vi "Update Connection Control.vi"(7 "Direction to Include":T1=enum."Publisher", 8 "error in (no error)":errorcluster, 10 "Channels":refnum<vi>, 11 "Channel Connection":refnum<vi>) -> (0 "error out":errorcluster)   [LabVIEW 2021, in "CIF_UI.lvclass"]
uses:
  CIF_UI.lvclass
  Typedef/Channel Connection.ctl
  Typedef/Direction to Include.ctl
  CIF_UI.lvclass/CIF_UI.ctl
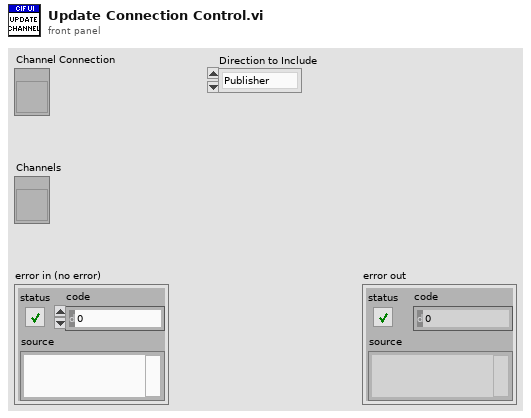
[diagram p1: front panel]
types:
  T1 = typedef "CIF_UI.lvclass/Direction to Include.ctl" = enum16{"All", "Subscriber", "Publisher"}
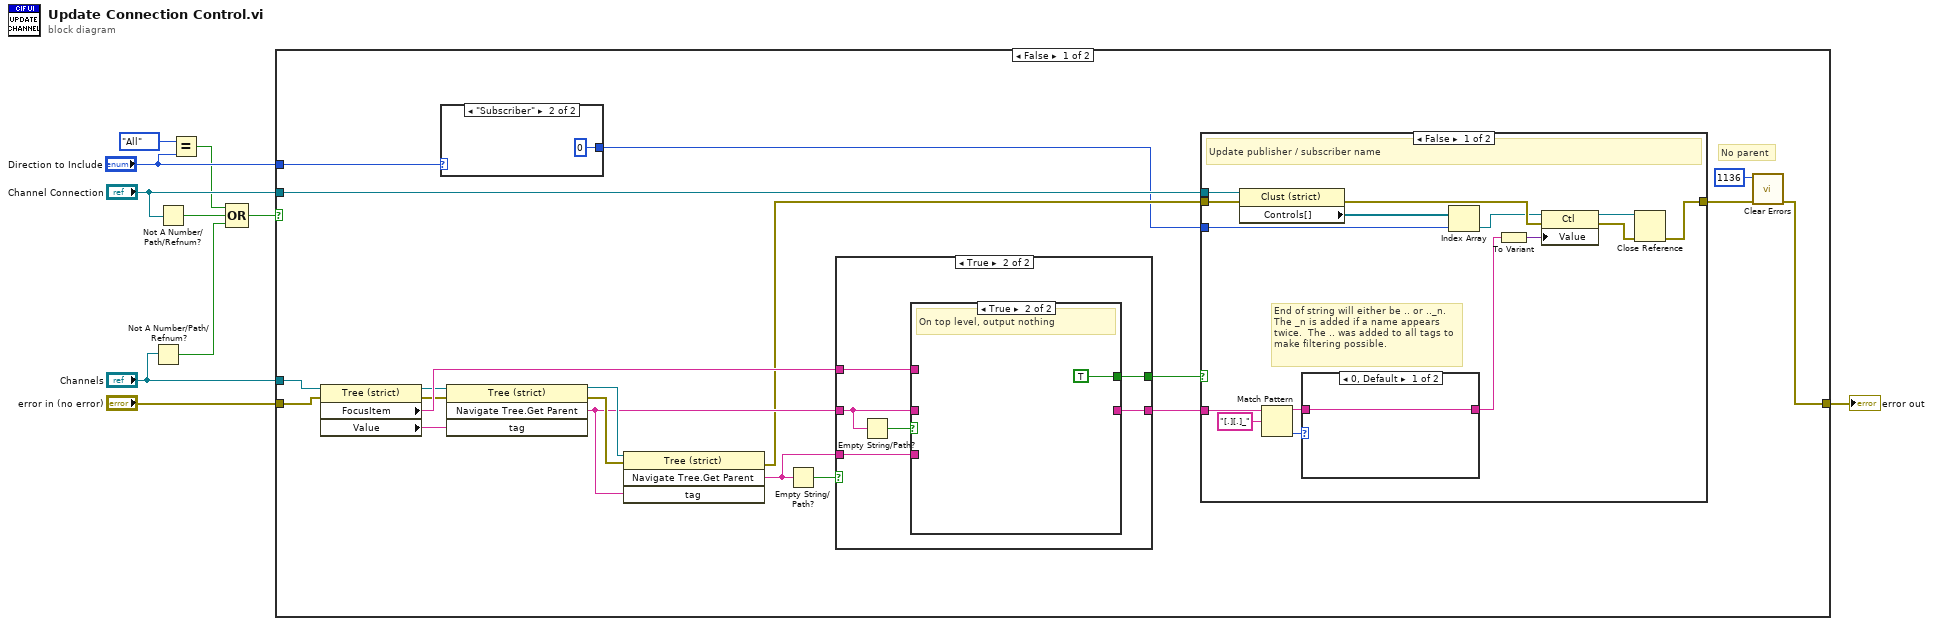
[diagram p0: block diagram]
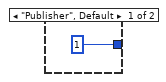
[diagram p2: hidden frame]
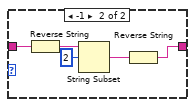
[diagram p3: hidden frame]
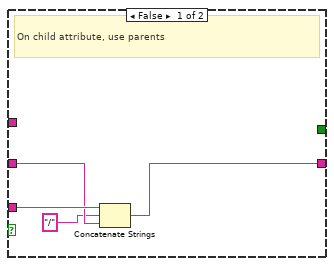
[diagram p5: hidden frame]
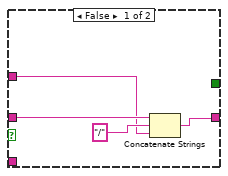
[diagram p6: hidden frame]
diagram:
  n1 = Not A Number/Path/Refnum?(number/path/refnum="Channels") -> (NaN/Path/Refnum?=w2:bool)
  n2 = Not A Number/Path/Refnum?(number/path/refnum="Channel Connection") -> (NaN/Path/Refnum?=w4:bool)
  n3 = Equal?(x=Direction_to_Include."All", y="Direction to Include") -> (x = y?=w3:bool)
  n4 = Compound Arithmetic op=OR(w3, w4, w2) -> (w1:bool)
  n5 = case shown="False" w1 {
    tunnel: "error in (no error)" -> [w24 w69]
    tunnel: [w16 w69] -> w9
    tunnel: "Channel Connection" -> [w14 _]
    tunnel: "Channels" -> [w13 _]
    tunnel: "Direction to Include" -> [w12 _]
    frame False {
      # "No parent"
      n6 = property class="Tree (strict)"(reference=w13, error in=w24) -> (error out=w26:errorcluster, "FocusItem"=w27:string, "Value"=w29:string)  [unwired: 1 out]
      n7 = case shown="\"Subscriber\"" w12 {
        tunnel: [1 ("index") 0 ("index")] -> w11
        frame "Publisher", Default {
        }
        frame "Subscriber" {
        }
      }
      n8 = invoke class="Tree (strict)" method="Navigate Tree.Get Parent"(reference=w13, error in=w26, "tag"=w29) -> (reference out=w23:refnum<vi>, error out=w22:errorcluster, "Navigate Tree:Get Parent"=w21:string)  [unwired: 1 in, 1 out]
      n9 = invoke class="Tree (strict)" method="Navigate Tree.Get Parent"(reference=w23, error in=w22, "tag"=w21) -> (error out=w18:errorcluster, "Navigate Tree:Get Parent"=w20:string)  [unwired: 1 in, 2 out]
      n10 = Empty String/Path?(string/path=w20) -> (empty?=w28:bool)
      n11 = case shown="True" w28 {
        tunnel: w21 -> [w56 w59]
        tunnel: w27 -> [_ w60]
        tunnel: [w54 w61] -> w25
        tunnel: w20 -> [w57 w58]
        tunnel: [_ w62] -> w19
        frame False {
          # "On child attribute, use parents"
          n12 = Concatenate Strings(w57, "/" ("string"), w56) -> (w54:string)
        }
        frame True {
          n13 = Empty String/Path?(string/path=w59) -> (empty?=w63:bool)
          n14 = case shown="True" w63 {
            tunnel: [_ TRUE] -> w62
            tunnel: [w64 _] -> w61
            tunnel: w60 -> [w65 _]
            tunnel: w59 -> [w66 _]
            tunnel: w58 -> [_ _]
            frame False {
              n15 = Concatenate Strings(w66, "/" ("string"), w65) -> (w64:string)
            }
            frame True {
              # "On top level, output nothing"
            }
          }
        }
      }
      n16 = case shown="False" w19 {
        tunnel: w25 -> [w36 _]
        tunnel: [w45 w53] -> w17
        tunnel: w14 -> [w44 _]
        tunnel: w18 -> [w38 w53]
        tunnel: w11 -> [w37 _]
        frame False {
          # "End of string will either be .. or .._n.  The _n is added if a name appears twice.  The .. was added to all tags to make filtering possible."
          # "Update publisher / subscriber name"
          n17 = property class="Clust (strict)"(reference=w44, error in=w38) -> (error out=w46:errorcluster, "Controls[]"=w40:refnum<vi>[])  [unwired: 1 out]
          n18 = Match Pattern(string=w36, regular expression="[.][.]_") -> (before substring=w33:string, offset past match=w34:i32)  [unwired: 1 in, 2 out]
          n19 = case shown="0, Default" w34 {
            tunnel: w33 -> [w47 w52]
            tunnel: [w47 w48] -> w32
            frame 0, Default {
            }
            frame -1 {
              n20 = Reverse String(1:w52) -> (0:w51:string)
              n21 = String Subset(string=w51, offset (0)=2) -> (substring=w49:string)  [unwired: 1 in]
              n22 = Reverse String(1:w49) -> (0:w48:string)
            }
          }
          n23 = Index Array(array=w40, index=w37) -> (element=w39:refnum<vi>)
          n24 = To Variant(anything=w32) -> (Variant=w43:variant)
          n25 = property class="Ctl"(reference=w39, error in=w46, "Value"=w43) -> (reference out=w42:refnum<vi>, error out=w41:errorcluster)
          n26 = Close Reference(reference=w42, error in (no error)=w41) -> (error out=w45:errorcluster)
        }
        frame True {
        }
      }
      n27 = call <vilib>:"Clear Errors.vi"("error in (no error)"=w17, "specific error code to clear (0: all)"=1136) -> ("error out"=w16:errorcluster)  [unwired: 4 in, 1 out]
    }
    frame True {
    }
  }
  "error out" <- w9
